vi "S2C_ExeScriptResultRoute.vi"(7 "Q_Ref":refnum<queue>, 8 "Error In":errorcluster, 9 "LastMeas?":bool, 10 "Result":T1, 11 "Data In":string[][](array[string])) -> (0 "Error Out":errorcluster)   [LabVIEW 2015]
doc: "Update the results cell in the execution table for the currently executing line item, and determines the next step to take in the execution."
uses:
  Controls/S2C_ResultStatus.ctl
  Globals/S2C_Globals.vi
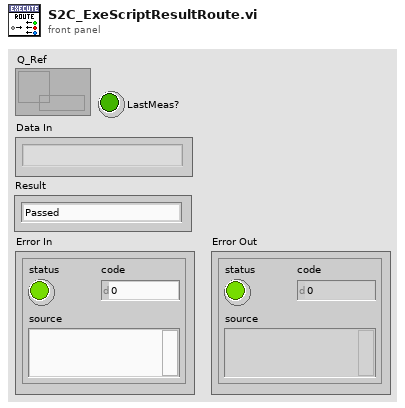
[diagram p1: front panel]
types:
  T1 = typedef "S2C_ResultStatus.ctl" = enum16{"Passed", "Failed", "Logged", "Aborted", "Error", "Testing...", "Paused", "No Record"}
  T2 = typedef "LVRowAndColumnUnsignedTypeDef.ctl" = cluster{"Row":u32, "Column":u32}
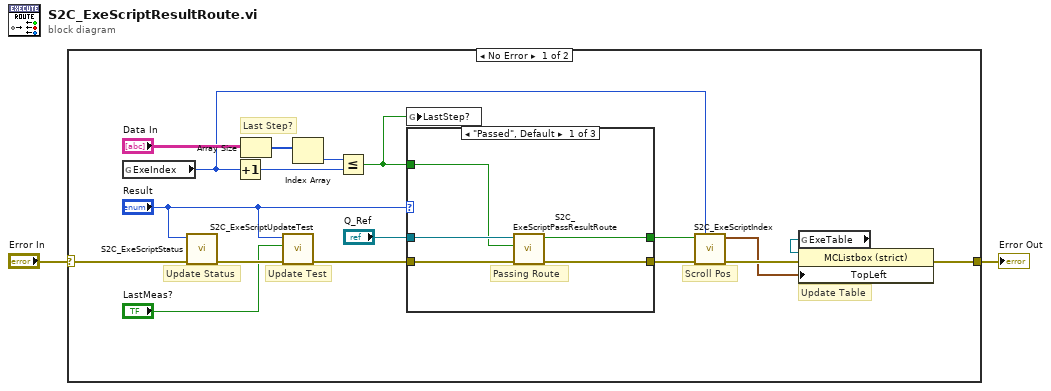
[diagram p0: block diagram]
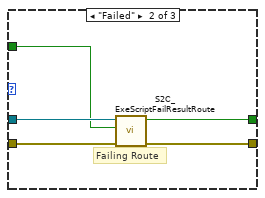
[diagram p2: hidden frame]
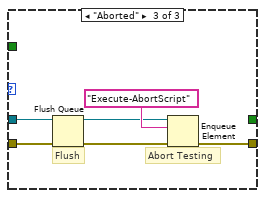
[diagram p3: hidden frame]
diagram:
  n1 = case shown="No Error" "Error In" {
    selector: "Error In" -> [w7 w36]
    tunnel: [w4 w36] -> w1
    frame No Error {
      # "Update Test"
      # "Update Status"
      # "Update Table"
      # "Scroll Pos"
      # "Last Step?"
      n2 = global read "S2C_Globals.vi" "ExeIndex"() -> (w3:i32)
      n3 = call "S2C_ExeScriptStatus.vi"("Status"="Result") -> ("Error Out"=w8:errorcluster)  [unwired: 10 in]
      n4 = Increment(x=w3) -> (x+1=w16:i32)
      n5 = Array Size(array="Data In") -> (size(s)=w18:i32[])
      n6 = call "S2C_ExeScriptUpdateTest.vi"("Error In"=w8, "LastMeas?"="LastMeas?", "Status"="Result") -> ()  [unwired: 8 in, 1 out]
      n7 = Index Array(array=w18) -> (element=w17:i32)  [unwired: 1 in]
      n8 = Less Or Equal?(x=w17, y=w16) -> (x <= y?=w15:bool)
      n9 = global write "S2C_Globals.vi" "LastStep?"(w15) -> ()
      n10 = case shown="\"Passed\", Default" "Result" {
        tunnel: w7 -> [w24 w29 w34]
        tunnel: [w23 w28 w33] -> w14
        tunnel: "Q_Ref" -> [w22 w27 w31]
        tunnel: w15 -> [w21 w26 _]
        tunnel: [w20 w25 _] -> w13
        frame "Passed", Default {
          # "Passing Route"
          n11 = call "S2C_ExeScriptPassResultRoute.vi"("Error In"=w24, "LastStep?"=w21, "Q_Ref"=w22) -> ("Error Out"=w23:errorcluster, "IncRow?"=w20:bool)  [unwired: 7 in]
        }
        frame "Failed" {
          # "Failing Route"
          n12 = call "S2C_ExeScriptFailResultRoute.vi"("Error In"=w29, "LastStep?"=w26, "Q_Ref"=w27) -> ("Error Out"=w28:errorcluster, "IncRow?"=w25:bool)  [unwired: 7 in]
        }
        frame "Aborted" {
          # "Flush"
          # "Abort Testing"
          n13 = Flush Queue(queue=w31, error in (no error)=w34) -> (queue out=w30:refnum<queue>, error out=w32:errorcluster)  [unwired: 1 out]
          n14 = Enqueue Element(queue=w30, element="Execute-AbortScript", error in (no error)=w32) -> (error out=w33:errorcluster)  [unwired: 1 in, 2 out]
        }
      }
      n15 = call "S2C_ExeScriptIndex.vi"("Index"=w3, "Error In"=w14, "IncRow?"=w13) -> ("Error Out"=w11:errorcluster, "TopCell Out"=w9:T2)  [unwired: 7 in]
      n16 = global read "S2C_Globals.vi" "ExeTable"() -> (w12:refnum<vi>)
      n17 = property class="MCListbox (strict)"(reference=w12, error in=w11, "TopLeft"=w9) -> (error out=w4:errorcluster)  [unwired: 1 out]
    }
    frame Error {
    }
  }
  "Error Out" <- w1
